vi "OpenConfigurationFile.vi"(8 "error in (no error)":errorcluster, 11 "GCMConfigurationManager in":refnum<class "GCMConfigurationManager.lvclass">) -> (0 "error out":errorcluster, 2 "FileRefnum":T1, 3 "GCMConfigurationManager out":refnum<class "GCMConfigurationManager.lvclass">)   [LabVIEW 2014, in "GCMConfigurationManager.lvclass"]
uses:
  GCMConfigurationManager.lvclass
  <vilib>/Utility/config.llb/Config Data RefNum.ctl
  GCMConfigurationManager.lvclass/GCMConfigurationManager.ctl
  <vilib>/Utility/config.llb/NI_LVConfig.lvlib
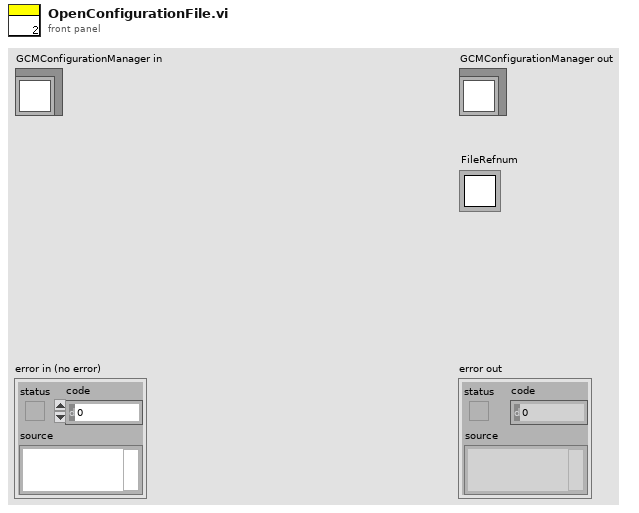
[diagram p1: front panel]
types:
  T1 = typedef "NI_LVConfig.lvlib/Config Data RefNum.ctl" = refnum<k1>
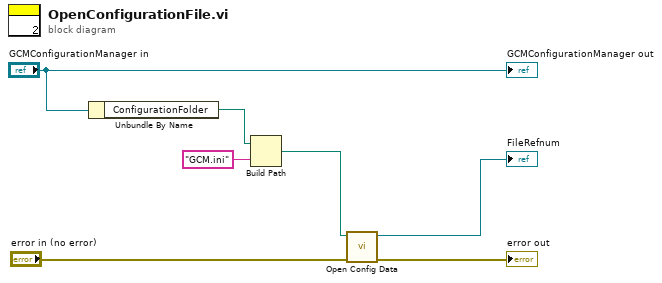
[diagram p0: block diagram]
diagram:
  n1 = Unbundle By Name("GCMConfigurationManager in") -> ("ConfigurationFolder"=w6:path)
  n2 = Build Path(base path=w6, name or relative path="GCM.ini") -> (appended path=w4:path)
  n3 = call <vilib>:"Open Config Data.vi"("error in (no error)"="error in (no error)", "configuration file path"=w4) -> ("error out"=→"error out":errorcluster, "refnum"=→"FileRefnum":T1)  [unwired: 7 in, 1 out]
  "GCMConfigurationManager out" <- "GCMConfigurationManager in"
